vi "Write Init VI Properties.vi"(8 "Error In":errorcluster, 10 "Initialization VI Properties":T1, 11 "Custom Device .NET Ref In":refnum<k24>) -> (0 "Error Out":errorcluster, 3 "Custom Device .NET Ref Out":refnum<k24>)   [LabVIEW 2019, in "VeriStand Custom Device XML Parser.lvlib"]
doc: "Writes the properties of the custom device initialization VI"
uses:
  VeriStand Custom Device XML Parser.lvlib
  NationalInstruments.VeriStand.XMLReader
  XML Controls/Initialization VI Properties.ctl
  XML Controls/Execution Types.ctl
  XML Controls/Path Cluster.ctl
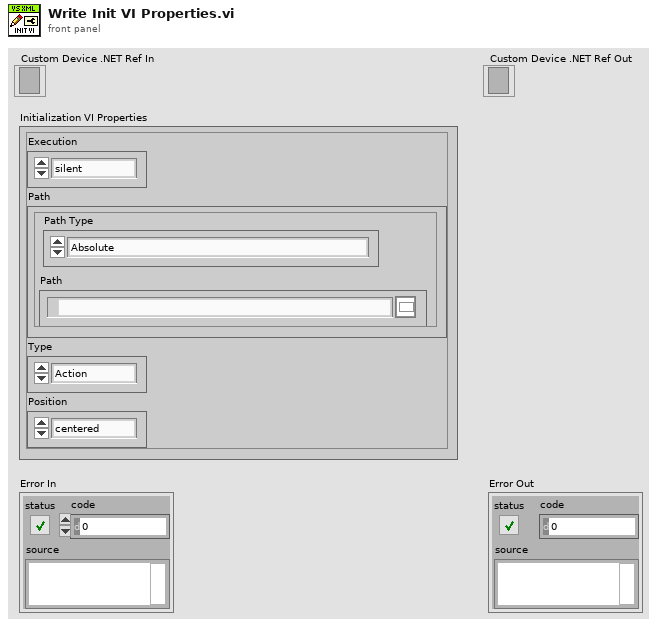
[diagram p1: front panel]
types:
  T1 = typedef "VeriStand Custom Device XML Parser.lvlib/Initialization VI Properties.ctl" = cluster{"Execution":T2, "Path":T3, "Type":enum16{"Action", "VI"}, "Position":enum16{"centered", "mouse pointer"}}
  T2 = typedef "VeriStand Custom Device XML Parser.lvlib/Execution Types.ctl" = enum16{"silent", "modal", "floating", "default"}
  T3 = typedef "VeriStand Custom Device XML Parser.lvlib/Path Cluster.ctl" = cluster{"Path":path, "Path Type":enum16{"Absolute", "To Base", "To Common Doc Dir", "To Application Data Dir"}}
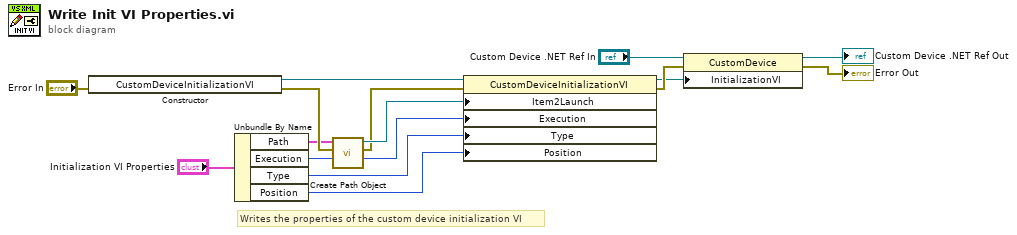
[diagram p0: block diagram]
diagram:
  # "Writes the properties of the custom device initialization VI"
  n1 = constructor class="CustomDeviceInitializationVI"(error in="Error In") -> (reference out=w7:refnum<k24>, error out=w4:errorcluster)  [unwired: 2 in, 1 out]
  n2 = Unbundle By Name("Initialization VI Properties") -> ("Path"=w3:T3, "Execution"=w8:T2, "Type"=w9:enum16{"Action", "VI"}, "Position"=w10:enum16{"centered", "mouse pointer"})
  n3 = call "Create Path Object.vi"("Error In"=w4, "Path Data Cluster"=w3) -> ("Error Out"=w1:errorcluster, "Path .NET Ref"=w2:refnum<k24>)  [unwired: 8 in]
  n4 = property class="CustomDeviceInitializationVI"(reference=w7, error in=w1, "Item2Launch"=w2, "Execution"=w8, "Type"=w9, "Position"=w10) -> (reference out=w12:refnum<k24>, error out=w13:errorcluster)
  n5 = property class="CustomDevice"(reference="Custom Device .NET Ref In", error in=w13, "InitializationVI"=w12) -> (reference out=→"Custom Device .NET Ref Out":refnum<k24>, error out=→"Error Out":errorcluster)
